vi "Proc RXed.vi"(8 "List in":string[](array[string]), 9 "MsgBox in":string, 10 "counter in":i32, 11 "data in":string) -> (0 "List out":string[](array[string]), 1 "MsgBox out":string, 2 "counter out":i32)   [LabVIEW 2012]
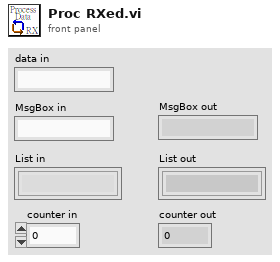
[diagram p1: front panel]
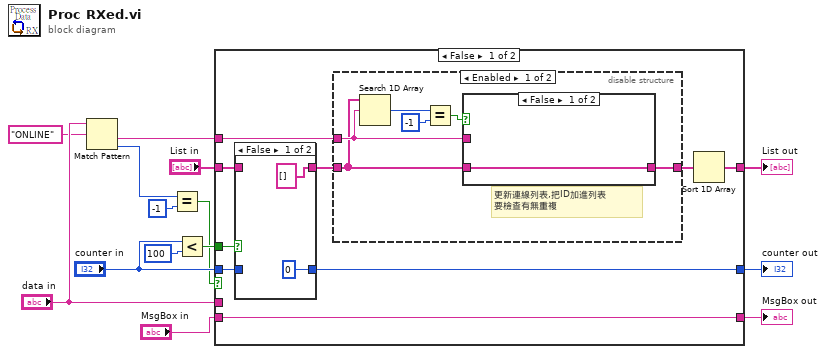
[diagram p0: block diagram]
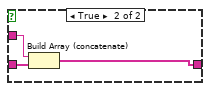
[diagram p2: hidden frame]
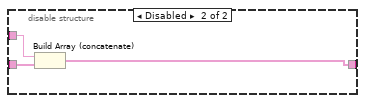
[diagram p3: hidden frame]
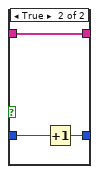
[diagram p4: hidden frame]
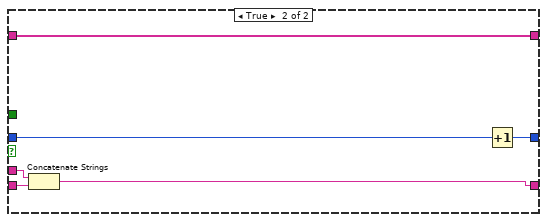
[diagram p5: hidden frame]
diagram:
  n1 = Match Pattern(string="data in", regular expression="ONLINE") -> (after substring=w5:string, offset past match=w4:i32)  [unwired: 1 in, 2 out]
  n2 = Equal?(x=w4, y=-1 ("offset (0)")) -> (x = y?=w3:bool)
  n3 = Less?(x="counter in", y=100) -> (x < y?=w9:bool)
  n4 = case shown="False" w3 {
    tunnel: "data in" -> [_ w45]
    tunnel: w5 -> [w23 _]
    tunnel: "counter in" -> [w19 w46]
    tunnel: [w22 w47] -> w6
    tunnel: w9 -> [w18 _]
    tunnel: [w17 w44] -> w11
    tunnel: "List in" -> [w16 w44]
    tunnel: "MsgBox in" -> [w15 w43]
    tunnel: [w15 w42] -> w14
    frame False {
      n5 = case shown="False" w18 {
        tunnel: [0 ("t") w41] -> w22
        tunnel: [string[] [] ("OnlineList") w39] -> w21
        tunnel: w19 -> [_ w40]
        tunnel: w16 -> [_ w39]
        frame False {
        }
        frame True {
          n6 = Increment(x=w40) -> (x+1=w41:i32)
        }
      }
      n7 = disable-structure shown="Enabled" {
        disable-tunnel: w23 -> [w26 w36]
        disable-tunnel: w21 -> [w25 w35]
        disable-tunnel: [w24 w34] -> w20
        frame Enabled {
          # "更新連線列表,把ID加進列表\n要檢查有無重複"
          n8 = Search 1D Array(1D array=w25, element=w26) -> (index of element=w27:i32)  [unwired: 1 in]
          n9 = Equal?(x=w27, y=-1) -> (x = y?=w28:bool)
          n10 = case shown="False" w28 {
            tunnel: [w30 w33] -> w24
            tunnel: w26 -> [_ w32]
            tunnel: w25 -> [w30 w31]
            frame False {
            }
            frame True {
              n11 = Build Array (concatenate)(w32, w31) -> (w33:string[])
            }
          }
        }
        frame Disabled {
          n12 = Build Array (concatenate)(w36, w35) -> (w34:string[])
        }
      }
      n13 = Sort 1D Array(array=w20) -> (sorted array=w17:string[])
    }
    frame True {
      n14 = Concatenate Strings(w45, w43) -> (w42:string)
      n15 = Increment(x=w46) -> (x+1=w47:i32)
    }
  }
  "MsgBox out" <- w14
  "List out" <- w11
  "counter out" <- w6
